vi "Get_dR.vi"(1 "[IN] dY":dbl, 2 "[IN] dX":dbl) -> (0 "[OUT] dR":dbl)   [LabVIEW 2017]
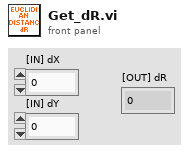
[diagram p1: front panel]
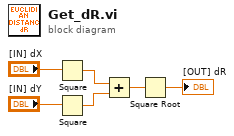
[diagram p0: block diagram]
diagram:
  n1 = Square(x="[IN] dX") -> (x^2=w4:dbl)
  n2 = Square(x="[IN] dY") -> (x^2=w3:dbl)
  n3 = Add(x=w4, y=w3) -> (x+y=w2:dbl)
  n4 = Square Root(x=w2) -> (sqrt(x)=→"[OUT] dR":dbl)
